vi "cold_cathode_control.vi"(8 "data task error in":errorcluster, 10 "press task in":refnum<k21>, 11 "Cold Cathode Gauge Channel":tag="Dev3/ai6") -> (0 "press error out":errorcluster, 2 "press task out":refnum<k21>, 3 "Cold Cathode Gauge Pressure":dbl)   [LabVIEW 2014]
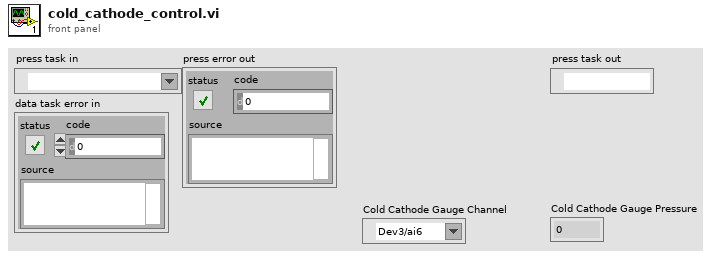
[diagram p1: front panel]
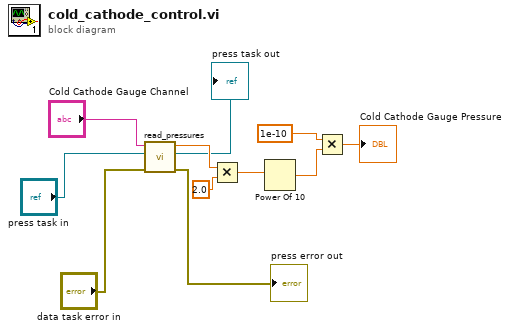
[diagram p0: block diagram]
diagram:
  n1 = call "read_pressures.vi"("data task error in"="data task error in", "press task in"="press task in", "Channel 1"="Cold Cathode Gauge Channel") -> ("press error out"=→"press error out":errorcluster, "press task out"=→"press task out":refnum<k21>, "Ch. 1 value"=w9:dbl)  [unwired: 6 in]
  n2 = Multiply(x=w9, y=2.0) -> (x*y=w7:dbl)
  n3 = Power Of 10(x=w7) -> (10^x=w10:dbl)
  n4 = Multiply(x=1e-10, y=w10) -> (x*y=→"Cold Cathode Gauge Pressure":dbl)
